vi "PM-share_error.vi"(8 "error in (no error)":errorcluster, 9 "module name":string, 11 "init_cluster":T1) -> (0 "error out":errorcluster)   [LabVIEW 2018]
uses:
  PM-init-data_cluster.ctl
  PM-init-user_events.ctl
  PM-common-heartrate_data.ctl
  PM-common-peak-detect_settings.ctl
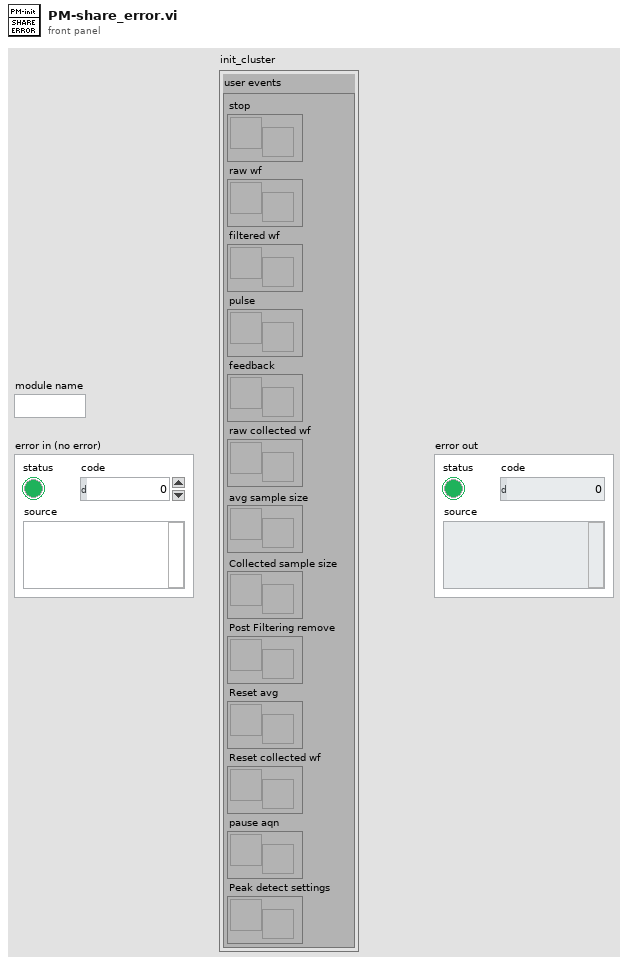
[diagram p1: front panel]
types:
  T1 = typedef "PM-init-data_cluster.ctl" = cluster{"user events":T2}
  T2 = typedef "PM-init-user_events.ctl" = cluster{"stop":refnum<user-event>, "raw wf":refnum<user-event>, "filtered wf":refnum<user-event>, "pulse":refnum<user-event>, "feedback":refnum<user-event>, "raw collected wf":refnum<user-event>, "avg sample size":refnum<user-event>, "Collected sample size":refnum<user-event>, "Post Filtering remove":refnum<user-event>, "Reset avg":refnum<user-event>, "Reset collected wf":refnum<user-event>, "pause aqn":refnum<user-event>, "Peak detect settings":refnum<user-event>}
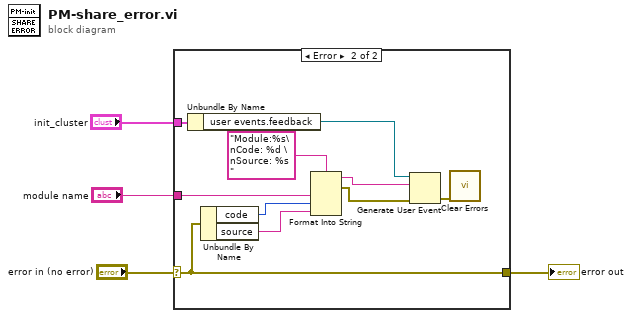
[diagram p0: block diagram]
diagram:
  n1 = case shown="Error" "error in (no error)" {
    selector: "error in (no error)" -> [w5 w6]
    tunnel: "init_cluster" -> [_ w15]
    tunnel: "module name" -> [_ w9]
    tunnel: [w5 w6] -> w1
    frame No Error {
    }
    frame Error {
      n2 = Unbundle By Name(w15) -> ("user events.feedback"=w14:refnum<user-event>)
      n3 = Unbundle By Name(w6) -> ("code"=w10:i32, "source"=w11:string)
      n4 = Format Into String(format string="Module:%s\nCode: %d \nSource: %s ", w9, w10, w11) -> (resulting string=w8:string, error out=w7:errorcluster)  [unwired: 2 in]
      n5 = Generate User Event(user event=w14, event data cluster=w8, error in=w7) -> (error out=w13:errorcluster)  [unwired: 1 in, 1 out]
      n6 = call <vilib>:"Clear Errors.vi"("error in (no error)"=w13) -> ()  [unwired: 5 in, 2 out]
    }
  }
  "error out" <- w1
